vi "Write Time Info Msg.vi"(10 "Timer.lvlib:Time Info Msg.lvclass":refnum<class "Time Info Msg.lvclass">, 11 "Timer in":refnum<class "Timer.lvclass">) -> (3 "Timer out":refnum<class "Timer.lvclass">)   [LabVIEW 2019, in "Timer.lvlib" / "Timer.lvclass"]
uses:
  Timer.lvclass
  Timer Messages/Time Info Msg/Time Info Msg.lvclass
  Timer.lvclass/Timer.ctl
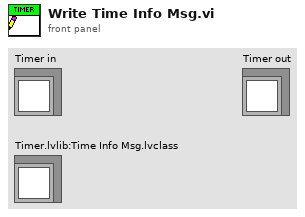
[diagram p1: front panel]
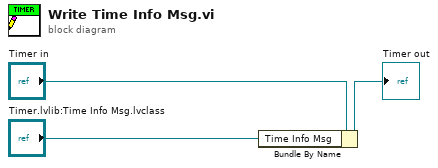
[diagram p0: block diagram]
diagram:
  n1 = Bundle By Name(cluster="Timer in", "Time Info Msg"="Timer.lvlib:Time Info Msg.lvclass") -> (→"Timer out":refnum<class "Timer.lvclass">)
